vi "Configure Trigger for Source.vi"(8 "error in (no error)":errorcluster, 11 "Reference values":T1={"dcpower session reservation"=refnum, "Source handle array"=[], "Source channel name array"=[], "Load handle"="", "Load channel name"="", "Source voltage values"=[], "Load current values"=[], "Number of steps"=0, "Source sequence name"="", "Source terminal name"="", "Measure terminal name"="", "scope session reservation"=refnum, "Scope handles"=[], "connection map"={}, "instrument info map array"=[], "Enable TClk"=FALSE, "dmm session reservation"=refnum, "dmm handle array"=[], "DMM Trigger Source"=enum."Immediate", "DMM Sample Trigger"=enum."TTL 0", "Measurement Results"={"Status"="", "Voltage values"=[], "Source sweep points"=0, "Load sweep points"=0, "Source voltages"=[], "Source currents"=[], "Load voltages"=[], "Load currents"=[], "Load voltage deviation"=[], "Efficiency"=[], "Maximum efficiency"=[], "Minimum load voltage"=[], "Maximum load voltage"=[], "Minimum load regulation"=[], "Maximum load regulation"=[], "waveform pins"=[], "waveform sites"=[], "waveform t0 array"=[], "waveform dt array"=[], "waveform length array"=[], "concatenated waveform Y"=[]}, "Additional measurements"={"voltage measurements from all sources"=[], "current measurements from all sources"=[], "all dmm measurements"=[], "all scope waverforms"=[]}}) -> (0 "error out":errorcluster, 3 "Reference values out":T1={"dcpower session reservation"=refnum, "Source handle array"=[], "Source channel name array"=[], "Load handle"="", "Load channel name"="", "Source voltage values"=[], "Load current values"=[], "Number of steps"=0, "Source sequence name"="", "Source terminal name"="", "Measure terminal name"="", "scope session reservation"=refnum, "Scope handles"=[], "connection map"={}, "instrument info map array"=[], "Enable TClk"=FALSE, "dmm session reservation"=refnum, "dmm handle array"=[], "DMM Trigger Source"=enum."Immediate", "DMM Sample Trigger"=enum."TTL 0", "Measurement Results"={"Status"="", "Voltage values"=[], "Source sweep points"=0, "Load sweep points"=0, "Source voltages"=[], "Source currents"=[], "Load voltages"=[], "Load currents"=[], "Load voltage deviation"=[], "Efficiency"=[], "Maximum efficiency"=[], "Minimum load voltage"=[], "Maximum load voltage"=[], "Minimum load regulation"=[], "Maximum load regulation"=[], "waveform pins"=[], "waveform sites"=[], "waveform t0 array"=[], "waveform dt array"=[], "waveform length array"=[], "concatenated waveform Y"=[]}, "Additional measurements"={"voltage measurements from all sources"=[], "current measurements from all sources"=[], "all dmm measurements"=[], "all scope waverforms"=[]}})   [LabVIEW 2021, in "Efficiency And Load Regulation with Pin Map.lvlib"]
uses:
  Efficiency And Load Regulation with Pin Map.lvlib
  Reference values.ctl
  <vilib>/Plug-In SDKs/Clients/Session Management V1/Session Reservation/Session Reservation.lvclass
  common/Instrument Control/Scope/TClk/Instrument Info.ctl
  common/Instrument Control/Scope Parameters.ctl
  <instrlib>/niScope/Controls/niScope vertical coupling.ctl
  <instrlib>/niDMM/nidmm.llb/niDMM Trigger.ctl
  <instrlib>/niDMM/nidmm.llb/niDMM Sample Trigger.ctl
  Measurement Results.ctl
  Additional measurements.ctl
  <instrlib>/niDCPower/nidcpower.llb/niDCPower Configure Digital Edge Start Trigger With Channels.vi
  <instrlib>/niDCPower/nidcpower.llb/niDCPower Configure Digital Edge Source Trigger With Channels.vi
  <instrlib>/niDCPower/nidcpower.llb/niDCPower Disable Start Trigger With Channels.vi
  <instrlib>/niDCPower/nidcpower.llb/niDCPower Configure Digital Edge Measure Trigger With Channels.vi
  common/PMIC Common.lvlib
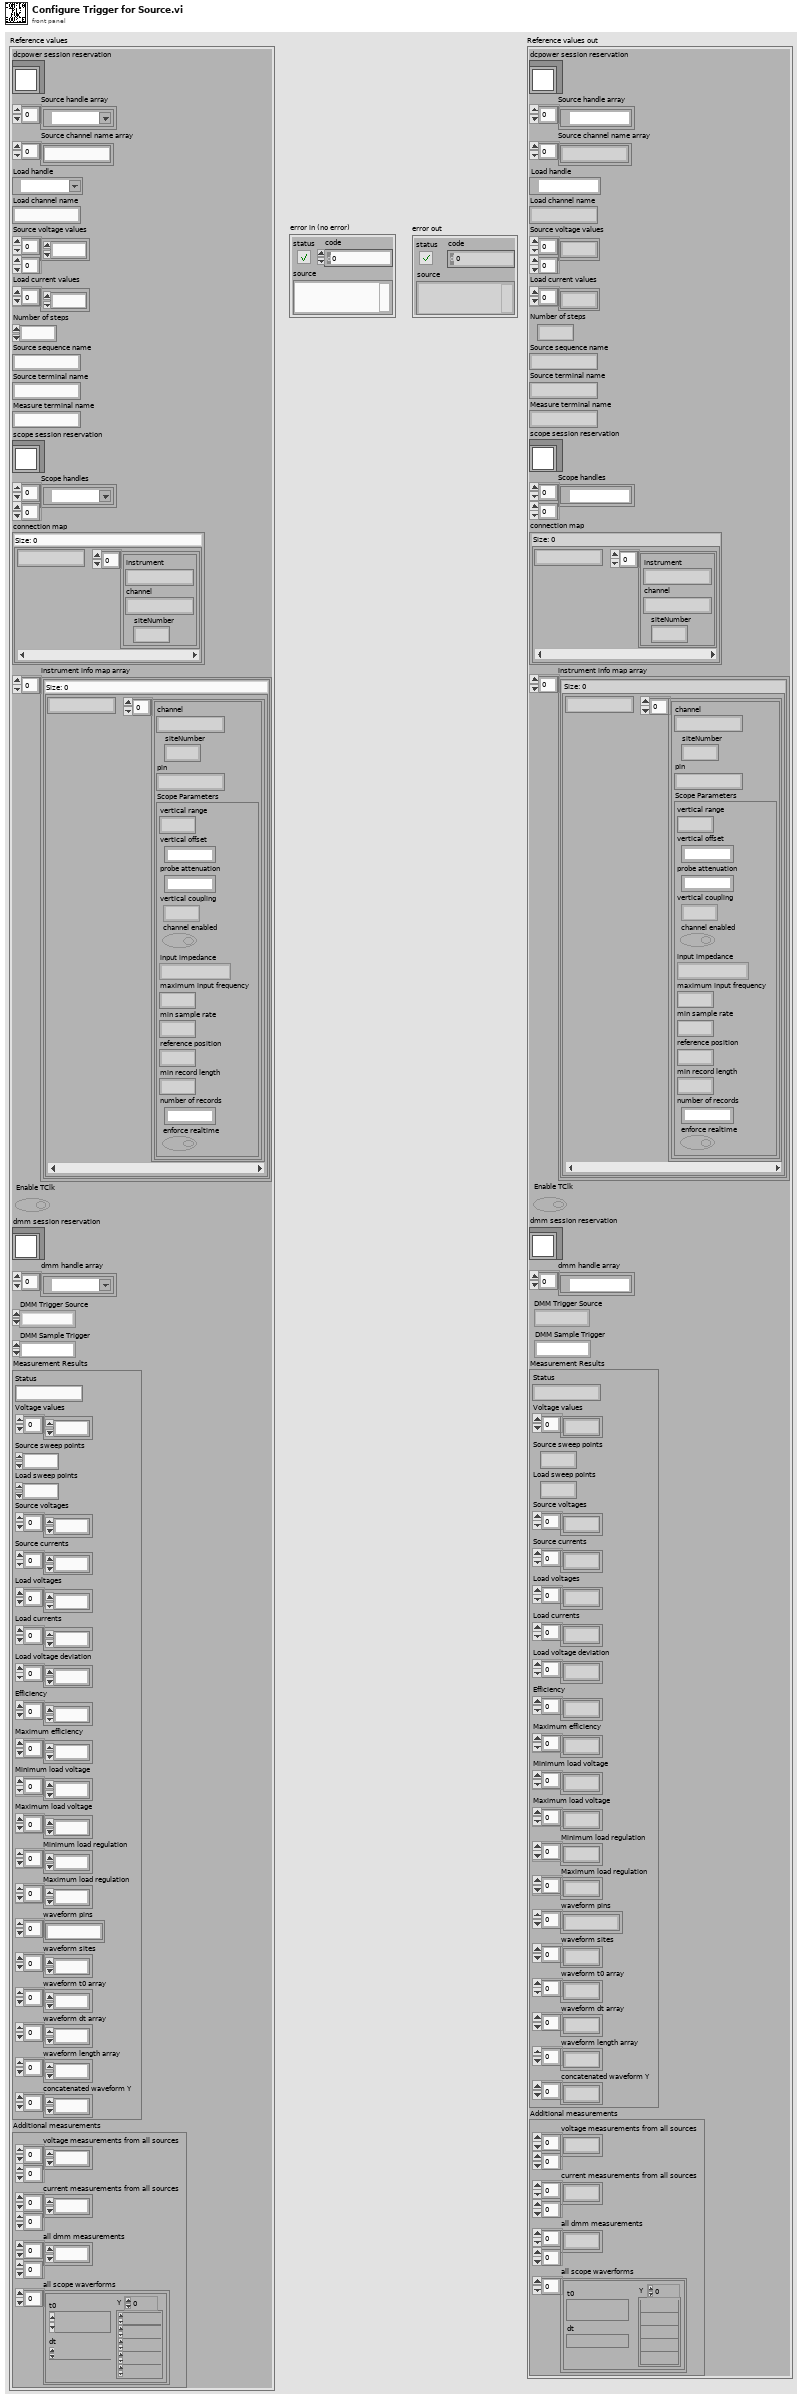
[diagram p1: front panel]
types:
  T1 = typedef "Efficiency And Load Regulation with Pin Map.lvlib/Reference values.ctl" = cluster{"dcpower session reservation":refnum<class "Session Reservation.lvclass">, "Source handle array":refnum<k15>[], "Source channel name array":string[], "Load handle":refnum<k15>, "Load channel name":string, "Source voltage values":dbl[][], "Load current values":dbl[], "Number of steps":i32, "Source sequence name":string, "Source terminal name":string, "Measure terminal name":string, "scope session reservation":refnum<class "Session Reservation.lvclass">, "Scope handles":refnum<k15>[][], "connection map":map{string, T2[]}, "instrument info map array":map{string, cluster{"channel":string, "siteNumber":i32, "pin":string, "Scope Parameters":T3}[]}[], "Enable TClk":bool, "dmm session reservation":refnum<class "Session Reservation.lvclass">, "dmm handle array":refnum<k15>[], "DMM Trigger Source":T5, "DMM Sample Trigger":T6, "Measurement Results":T7, "Additional measurements":T8}
  T2 = typedef "PMIC Common.lvlib/Instrument Info.ctl" = cluster{"instrument":string, "channel":string, "siteNumber":i32}
  T3 = typedef "PMIC Common.lvlib/Scope Parameters.ctl" = cluster{"vertical range":dbl, "vertical offset":dbl, "probe attenuation":dbl, "vertical coupling":T4, "channel enabled":bool, "input impedance":u32, "maximum input frequency":dbl, "min sample rate":dbl, "reference position":dbl, "min record length":i32, "number of records":i32, "enforce realtime":bool}
  T4 = typedef "niScope vertical coupling.ctl" = i32
  T5 = typedef "niDMM Trigger.ctl" = enum16{"Immediate", "External", "TTL 0", "TTL 1", "TTL 2", "TTL 3", "TTL 4", "TTL 5", "TTL 6", "Software", "TTL 7", "PXI Star", "LBR Trig 1", "Aux Trig 1"}
  T6 = typedef "niDMM Sample Trigger.ctl" = enum16{"Immediate", "External", "TTL 0", "TTL 1", "TTL 2", "TTL 3", "TTL 4", "TTL 5", "TTL 6", "Interval", "Software", "TTL 7", "PXI Star", "LBR Trig 1", "Aux Trig 1"}
  T7 = typedef "Efficiency And Load Regulation with Pin Map.lvlib/Measurement Results.ctl" = cluster{"Status":string, "Voltage values":dbl[], "Source sweep points":i32, "Load sweep points":i32, "Source voltages":dbl[], "Source currents":dbl[], "Load voltages":dbl[], "Load currents":dbl[], "Load voltage deviation":dbl[], "Efficiency":dbl[], "Maximum efficiency":dbl[], "Minimum load voltage":dbl[], "Maximum load voltage":dbl[], "Minimum load regulation":dbl[], "Maximum load regulation":dbl[], "waveform pins":string[], "waveform sites":i32[], "waveform t0 array":dbl[], "waveform dt array":dbl[], "waveform length array":i32[], "concatenated waveform Y":dbl[]}
  T8 = typedef "Efficiency And Load Regulation with Pin Map.lvlib/Additional measurements.ctl" = cluster{"voltage measurements from all sources":dbl[][], "current measurements from all sources":dbl[][], "all dmm measurements":dbl[][], "all scope waverforms":waveform(dbl)[]}
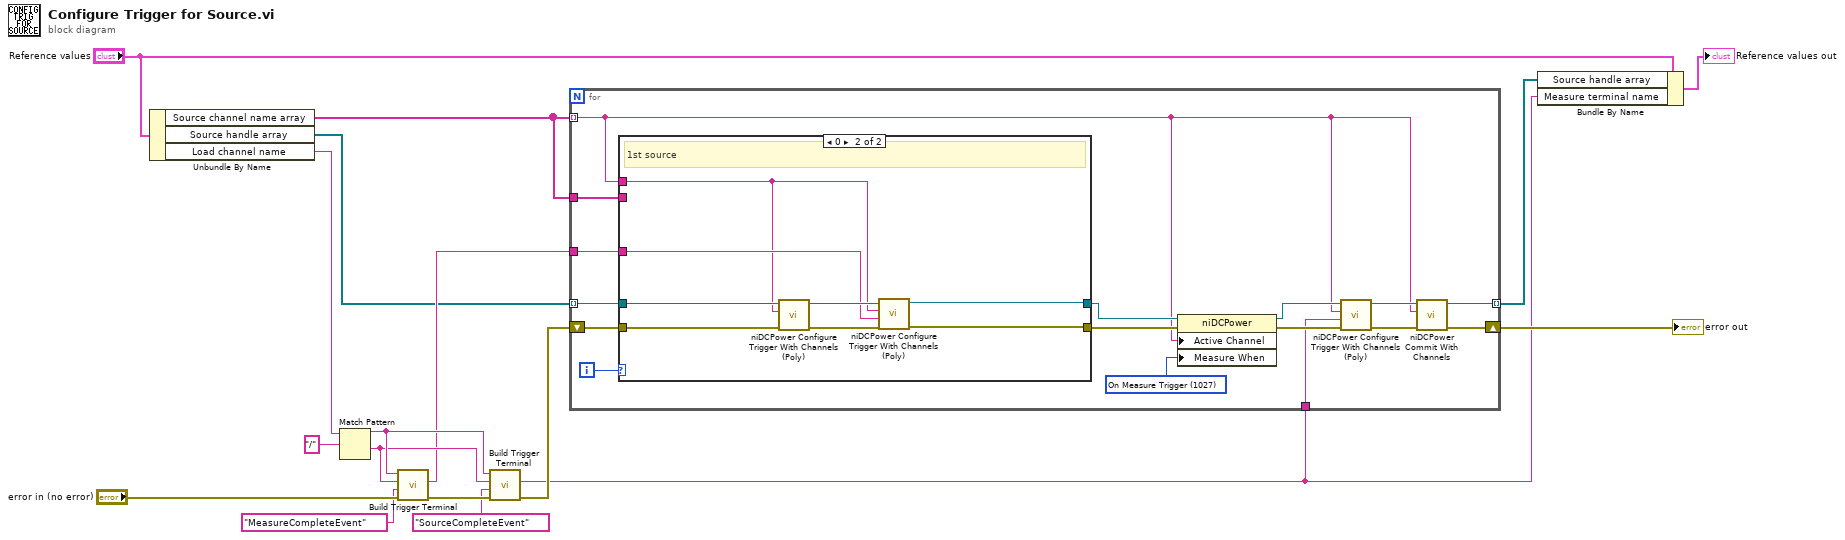
[diagram p0: block diagram]
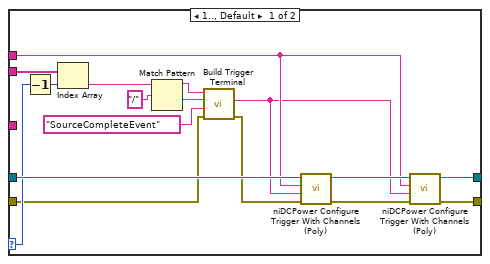
[diagram p2: hidden frame]
diagram:
  n1 = Unbundle By Name("Reference values") -> ("Source channel name array"=w16:string[], "Source handle array"=w2:refnum<k15>[], "Load channel name"=w12:string)
  n2 = Match Pattern(string=w12, regular expression="/") -> (before substring=w7:string, after substring=w6:string)  [unwired: 1 in, 2 out]
  n3 = call "Build Trigger Terminal.vi"("error in (no error)"="error in (no error)", "Trigger/Event Name"="MeasureCompleteEvent", "Channel Name"=w6, "Resource Name"=w7) -> ("error out"=w10:errorcluster, "Terminal Name"=w3:string)  [unwired: 6 in]
  n4 = call "Build Trigger Terminal.vi"("error in (no error)"=w10, "Trigger/Event Name"="SourceCompleteEvent", "Channel Name"=w6, "Resource Name"=w7) -> ("error out"=w9:errorcluster, "Terminal Name"=w8:string)  [unwired: 6 in]
  n5 = for {
    tunnel: w8 -> [w29]
    tunnel: w2 -> [w28] mode=indexing
    tunnel: w16 -> [w18] mode=indexing
    shift-right: [w25] -> w15
    shift-left: w9 -> [w26]
    tunnel: w16 -> [w22]
    tunnel: w3 -> [w21]
    tunnel: [w20] -> w1 mode=indexing
    i -> [w27]
    w19 = 1027 items=["Automatically after Source Complete"=1025, "On Demand"=1026, "On Measure Trigger"=1027] ("Measurement:Advanced:Measure When")
    n6 = case shown="0" w27 {
      selector: w27 -> [w42 _]
      tunnel: [w46 w53] -> w23
      tunnel: [w48 w55] -> w24
      tunnel: w28 -> [w50 w58]
      tunnel: w18 -> [w45 w51]
      tunnel: w26 -> [w36 w57]
      tunnel: w22 -> [w44 _]
      tunnel: w21 -> [_ w52]
      frame 1.., Default {
        n7 = Decrement(x=w42) -> (x-1=w43:i32)
        n8 = Index Array(array=w44, index=w43) -> (element=w40:string)
        n9 = Match Pattern(string=w40, regular expression="/") -> (before substring=w39:string, after substring=w38:string)  [unwired: 1 in, 2 out]
        n10 = call "Build Trigger Terminal.vi"("error in (no error)"=w36, "Trigger/Event Name"="SourceCompleteEvent", "Channel Name"=w38, "Resource Name"=w39) -> ("error out"=w35:errorcluster, "Terminal Name"=w34:string)  [unwired: 6 in]
        n11 = call-poly <instrlib>:"niDCPower Configure Trigger With Channels (Poly).vi"("error in (no error)"=w35, "input terminal"=w34, "channel name"=w45, "instrument handle"=w50) -> ("error out"=w49:errorcluster, "instrument handle out"=w47:refnum<k15>)  [unwired: 6 in]
        n12 = call-poly <instrlib>:"niDCPower Configure Trigger With Channels (Poly).vi"("error in (no error)"=w49, "input terminal"=w34, "channel name"=w45, "instrument handle"=w47) -> ("error out"=w48:errorcluster, "instrument handle out"=w46:refnum<k15>)  [unwired: 6 in]
      }
      frame 0 {
        # "1st source"
        n13 = call-poly <instrlib>:"niDCPower Configure Trigger With Channels (Poly).vi"("error in (no error)"=w57, "channel name"=w51, "instrument handle"=w58) -> ("error out"=w56:errorcluster, "instrument handle out"=w54:refnum<k15>)  [unwired: 7 in]
        n14 = call-poly <instrlib>:"niDCPower Configure Trigger With Channels (Poly).vi"("error in (no error)"=w56, "input terminal"=w52, "channel name"=w51, "instrument handle"=w54) -> ("error out"=w55:errorcluster, "instrument handle out"=w53:refnum<k15>)  [unwired: 6 in]
      }
    }
    n15 = property class="niDCPower"(reference=w23, error in=w24, "Active Channel"=w18, "Measure When"=w19) -> (reference out=w31:refnum<k15>, error out=w30:errorcluster)
    n16 = call-poly <instrlib>:"niDCPower Configure Trigger With Channels (Poly).vi"("error in (no error)"=w30, "input terminal"=w29, "channel name"=w18, "instrument handle"=w31) -> ("error out"=w32:errorcluster, "instrument handle out"=w33:refnum<k15>)  [unwired: 6 in]
    n17 = call <instrlib>:"niDCPower Commit With Channels.vi"("error in (no error)"=w32, "channel name"=w18, "instrument handle"=w33) -> ("error out"=w25:errorcluster, "instrument handle out"=w20:refnum<k15>)  [unwired: 7 in]
  }
  "error out" <- w15
  n18 = Bundle By Name(cluster="Reference values", "Source handle array"=w1, "Measure terminal name"=w8) -> (→"Reference values out":T1)
